vi "DAQ_Intial.vi"(8 "error in":errorcluster, 11 "DEV":string="Dev1") -> (0 "error out":errorcluster, 3 "task out":refnum<k21>)   [LabVIEW 2015]
uses:
  <vilib>/DAQmx/configure/timing.llb/DAQmx Timing (Sample Clock).vi
  <vilib>/DAQmx/create/channels.llb/DAQmx Create Channel (AI-Voltage-Basic).vi
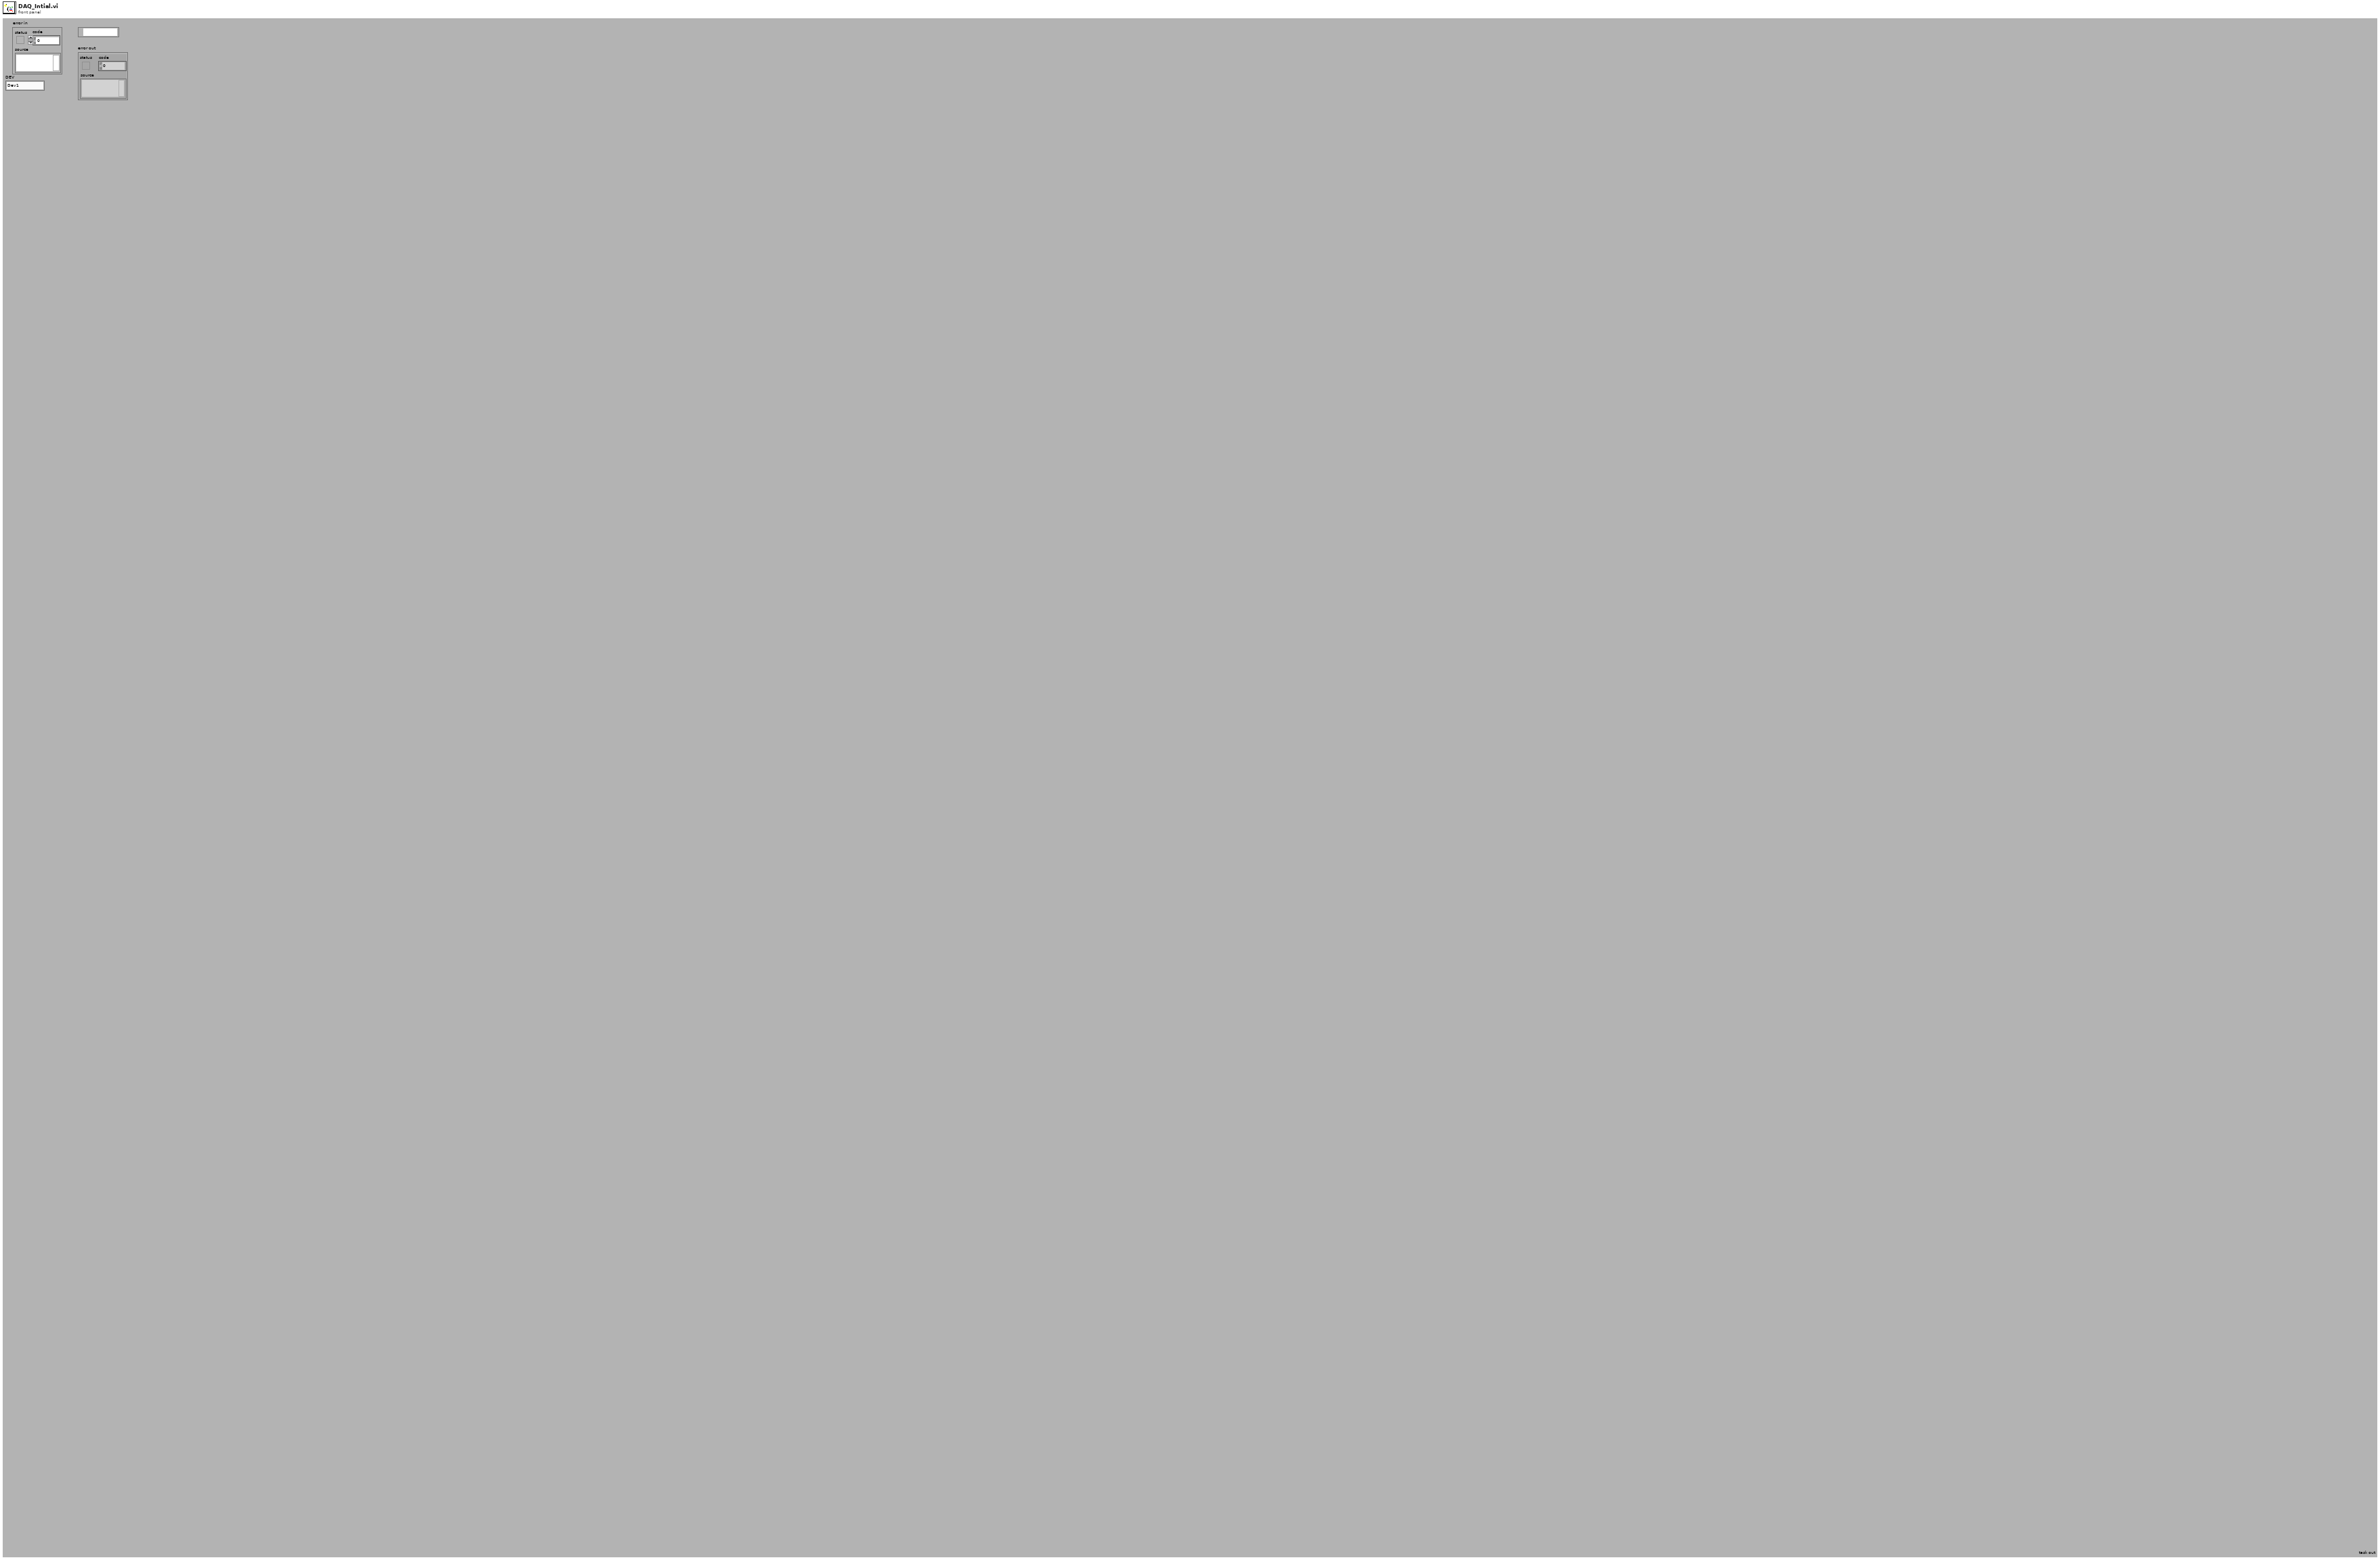
[diagram p1: front panel]
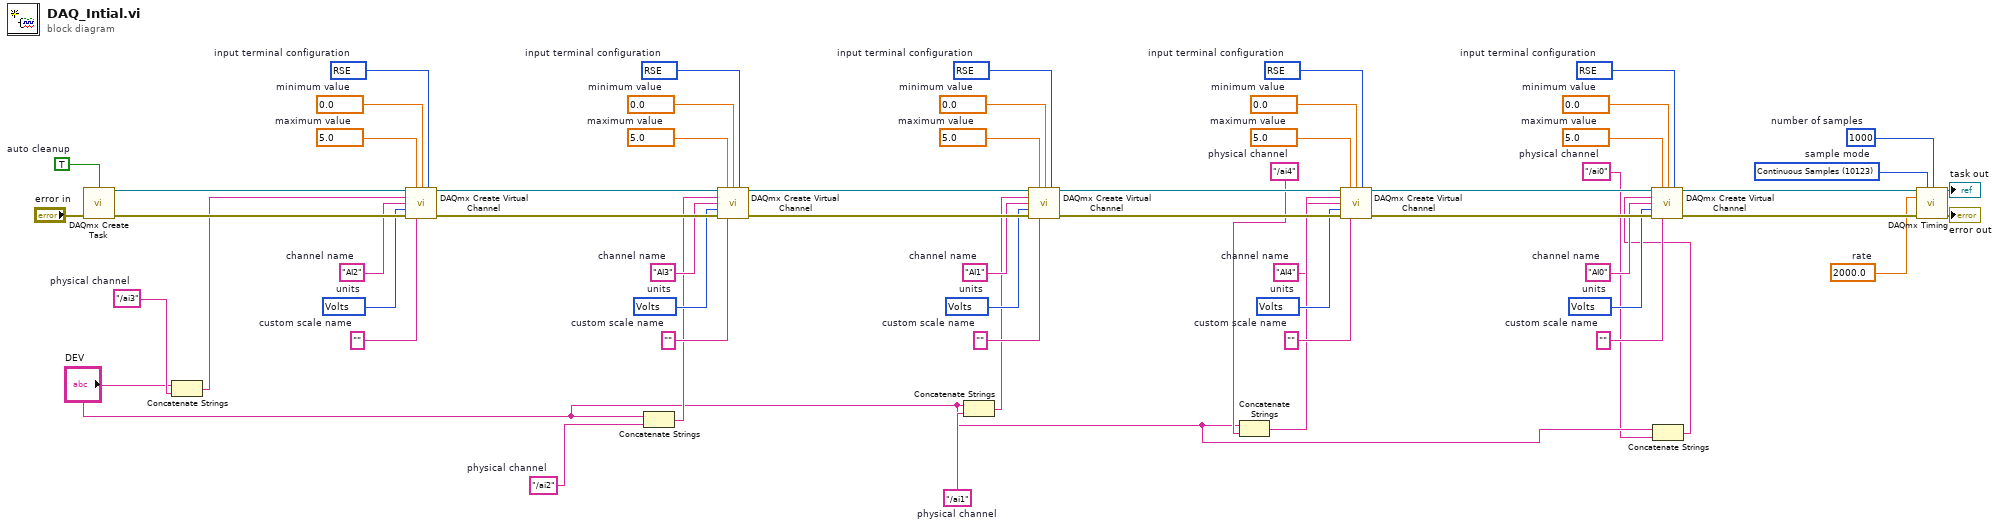
[diagram p0: block diagram]
diagram:
  w13 = 10123 items=["Finite Samples"=10178, "Continuous Samples"=10123, "Hardware Timed Single Point"=12522]  # sample mode
  w14 = 1000  # number of samples
  w15 = 2000.0  # rate
  w19 = 10083 items=["default"=-1, "RSE"=10083, "NRSE"=10078, "Differential"=10106, "Pseudodifferential"=12529]  # input terminal configuration
  w20 = 10348 items=["Volts"=10348, "From Custom Scale"=10065]  # units
  w21 = "AI0"  # channel name
  w23 = ""  # custom scale name
  w24 = 0.0  # minimum value
  w25 = 5.0  # maximum value
  w3 = "/ai0"  # physical channel
  w27 = 10083 items=["default"=-1, "RSE"=10083, "NRSE"=10078, "Differential"=10106, "Pseudodifferential"=12529]  # input terminal configuration
  w28 = 10348 items=["Volts"=10348, "From Custom Scale"=10065]  # units
  w1 = "AI4"  # channel name
  w30 = ""  # custom scale name
  w31 = 0.0  # minimum value
  w32 = 5.0  # maximum value
  w6 = "/ai4"  # physical channel
  w34 = 10083 items=["default"=-1, "RSE"=10083, "NRSE"=10078, "Differential"=10106, "Pseudodifferential"=12529]  # input terminal configuration
  w35 = 10348 items=["Volts"=10348, "From Custom Scale"=10065]  # units
  w36 = "AI1"  # channel name
  w38 = ""  # custom scale name
  w39 = 0.0  # minimum value
  w40 = 5.0  # maximum value
  w7 = "/ai1"  # physical channel
  w42 = 10083 items=["default"=-1, "RSE"=10083, "NRSE"=10078, "Differential"=10106, "Pseudodifferential"=12529]  # input terminal configuration
  w43 = 10348 items=["Volts"=10348, "From Custom Scale"=10065]  # units
  w44 = "AI3"  # channel name
  w46 = ""  # custom scale name
  w47 = 0.0  # minimum value
  w48 = 5.0  # maximum value
  w9 = "/ai2"  # physical channel
  w50 = 10083 items=["default"=-1, "RSE"=10083, "NRSE"=10078, "Differential"=10106, "Pseudodifferential"=12529]  # input terminal configuration
  w51 = 10348 items=["Volts"=10348, "From Custom Scale"=10065]  # units
  w52 = "AI2"  # channel name
  w54 = ""  # custom scale name
  w55 = 0.0  # minimum value
  w56 = 5.0  # maximum value
  w12 = "/ai3"  # physical channel
  w58 = TRUE  # auto cleanup
  n1 = call <vilib>:"DAQmx Create Task.vi"("auto cleanup"=w58, "error in"="error in") -> ("task out"=w57:refnum<k21>, "error out"=w59:errorcluster)  [unwired: 12 in]
  n2 = Concatenate Strings("DEV", w12) -> (w11:string)
  n3 = call-poly <vilib>:"DAQmx Create Virtual Channel.vi"("task in"=w57, "maximum value"=w56, "minimum value"=w55, "input terminal configuration"=w50, "physical channels"=w11, "name to assign"=w52, "units"=w51, "error in"=w59, "custom scale name"=w54) -> ("task out"=w49:refnum<k21>, "error out"=w53:errorcluster)  [unwired: 5 in]
  n4 = Concatenate Strings("DEV", w9) -> (w10:string)
  n5 = call-poly <vilib>:"DAQmx Create Virtual Channel.vi"("task in"=w49, "maximum value"=w48, "minimum value"=w47, "input terminal configuration"=w42, "physical channels"=w10, "name to assign"=w44, "units"=w43, "error in"=w53, "custom scale name"=w46) -> ("task out"=w41:refnum<k21>, "error out"=w45:errorcluster)  [unwired: 5 in]
  n6 = Concatenate Strings("DEV", w7) -> (w8:string)
  n7 = call-poly <vilib>:"DAQmx Create Virtual Channel.vi"("task in"=w41, "maximum value"=w40, "minimum value"=w39, "input terminal configuration"=w34, "physical channels"=w8, "name to assign"=w36, "units"=w35, "error in"=w45, "custom scale name"=w38) -> ("task out"=w33:refnum<k21>, "error out"=w37:errorcluster)  [unwired: 5 in]
  n8 = Concatenate Strings("DEV", w6) -> (w5:string)
  n9 = call-poly <vilib>:"DAQmx Create Virtual Channel.vi"("task in"=w33, "maximum value"=w32, "minimum value"=w31, "input terminal configuration"=w27, "physical channels"=w5, "name to assign"=w1, "units"=w28, "error in"=w37, "custom scale name"=w30) -> ("task out"=w26:refnum<k21>, "error out"=w29:errorcluster)  [unwired: 5 in]
  n10 = Concatenate Strings("DEV", w3) -> (w2:string)
  n11 = call-poly <vilib>:"DAQmx Create Virtual Channel.vi"("task in"=w26, "maximum value"=w25, "minimum value"=w24, "input terminal configuration"=w19, "physical channels"=w2, "name to assign"=w21, "units"=w20, "error in"=w29, "custom scale name"=w23) -> ("task out"=w16:refnum<k21>, "error out"=w22:errorcluster)  [unwired: 5 in]
  n12 = call-poly <vilib>:"DAQmx Timing.vi"("task/channels in"=w16, "sample mode"=w13, "samples per channel"=w14, "rate"=w15, "error in"=w22) -> ("task out"=→"task out":refnum<k21>, "error out"=→"error out":errorcluster)  [unwired: 9 in]
